vi "fpga_transmission_control_3V17.vi"() -> ()   [LabVIEW 2017]
doc: "3V15"
uses:
  Control 1.ctl
  <vilib>/Platform/TimedLoop/XDataNode/timing_clust.ctl
  <vilib>/Platform/TimedLoop/XDataNode/nitl_modes.ctl
  <vilib>/Platform/TimedLoop/XDataNode/wakeup.ctl
  <vilib>/Utility/config.llb/Read Key (String).vi
  <vilib>/Utility/config.llb/Write Key (String).vi
  <vilib>/Instr/_visa.llb/VISA Configure Serial Port (Serial Instr).vi
  <vilib>/platform/TimedLoop/XDataNode/XDataNode.xnode
  <vilib>/Platform/TimedLoop/XDataNode/XDNodeRunTimeDep.lvlib
  <vilib>/Utility/config.llb/NI_LVConfig.lvlib
  <vilib>/Analysis/NI_AALPro.lvlib
panel:
  in  "Tab Control":T1(tab)
  in  "Start":bool
  in  "Stop Program":bool
  out "Read":bool
  out "Sign":bool
  out "PWM":bool
  out "Output":bool
  out "Progress":dbl(slide) scale=0.0..100.0
  out "Time":dbl(slide) scale=0.0..100.0
  out "Timing":u32
  out "Timeslot":i32
  out "Timer":u32
  out "currentType":string
  out "Int_pixel":i16
  out "x-y":u16
  out "AD_Value":i16
  out "Complete Time":u32
  out "Kombi Chart":cluster{u16, i16}(graph)
  out "Histogram Graph":cluster{"Axis":dbl[], dbl[]}(graph)
  in  "fileName":string
  in  "pwmDtc":u8(slide)=25 scale=1.0..100.0
  in  "ExperimentalMetadata":T2
  in  "Fly":T3
  in  "Array":T5(array[cluster]) {"duration" step=1}
  in  "Path":path
  in  "VISA resource name":refnum<visa-resource-name>
  in  "LoadExperiment":bool
  in  "SaveExperiment":bool
  in  "ClearSetup":bool
  in  "Experimenter":T6
  in  "LoadMetadata":bool
  in  "SaveMetadata":bool
  in  "ClearMetaData":bool
  in  "URIs":T7
  out "VI Description":string
  out "outcome":u32
  in  "error in (no error)":errorcluster
  out "pattern":u32
  out "type":string
  out "contingency":string
  out "deleted portion":u8[](array[numeric])
  out "data":bool
  out "Error String":string
  out "error out":errorcluster
  in  "millisecond timer value 2":u32
  # "Universität Regensburg Elektronikwerkstatt Biologie/ VKL\n\njohann.schmid@ur.de"
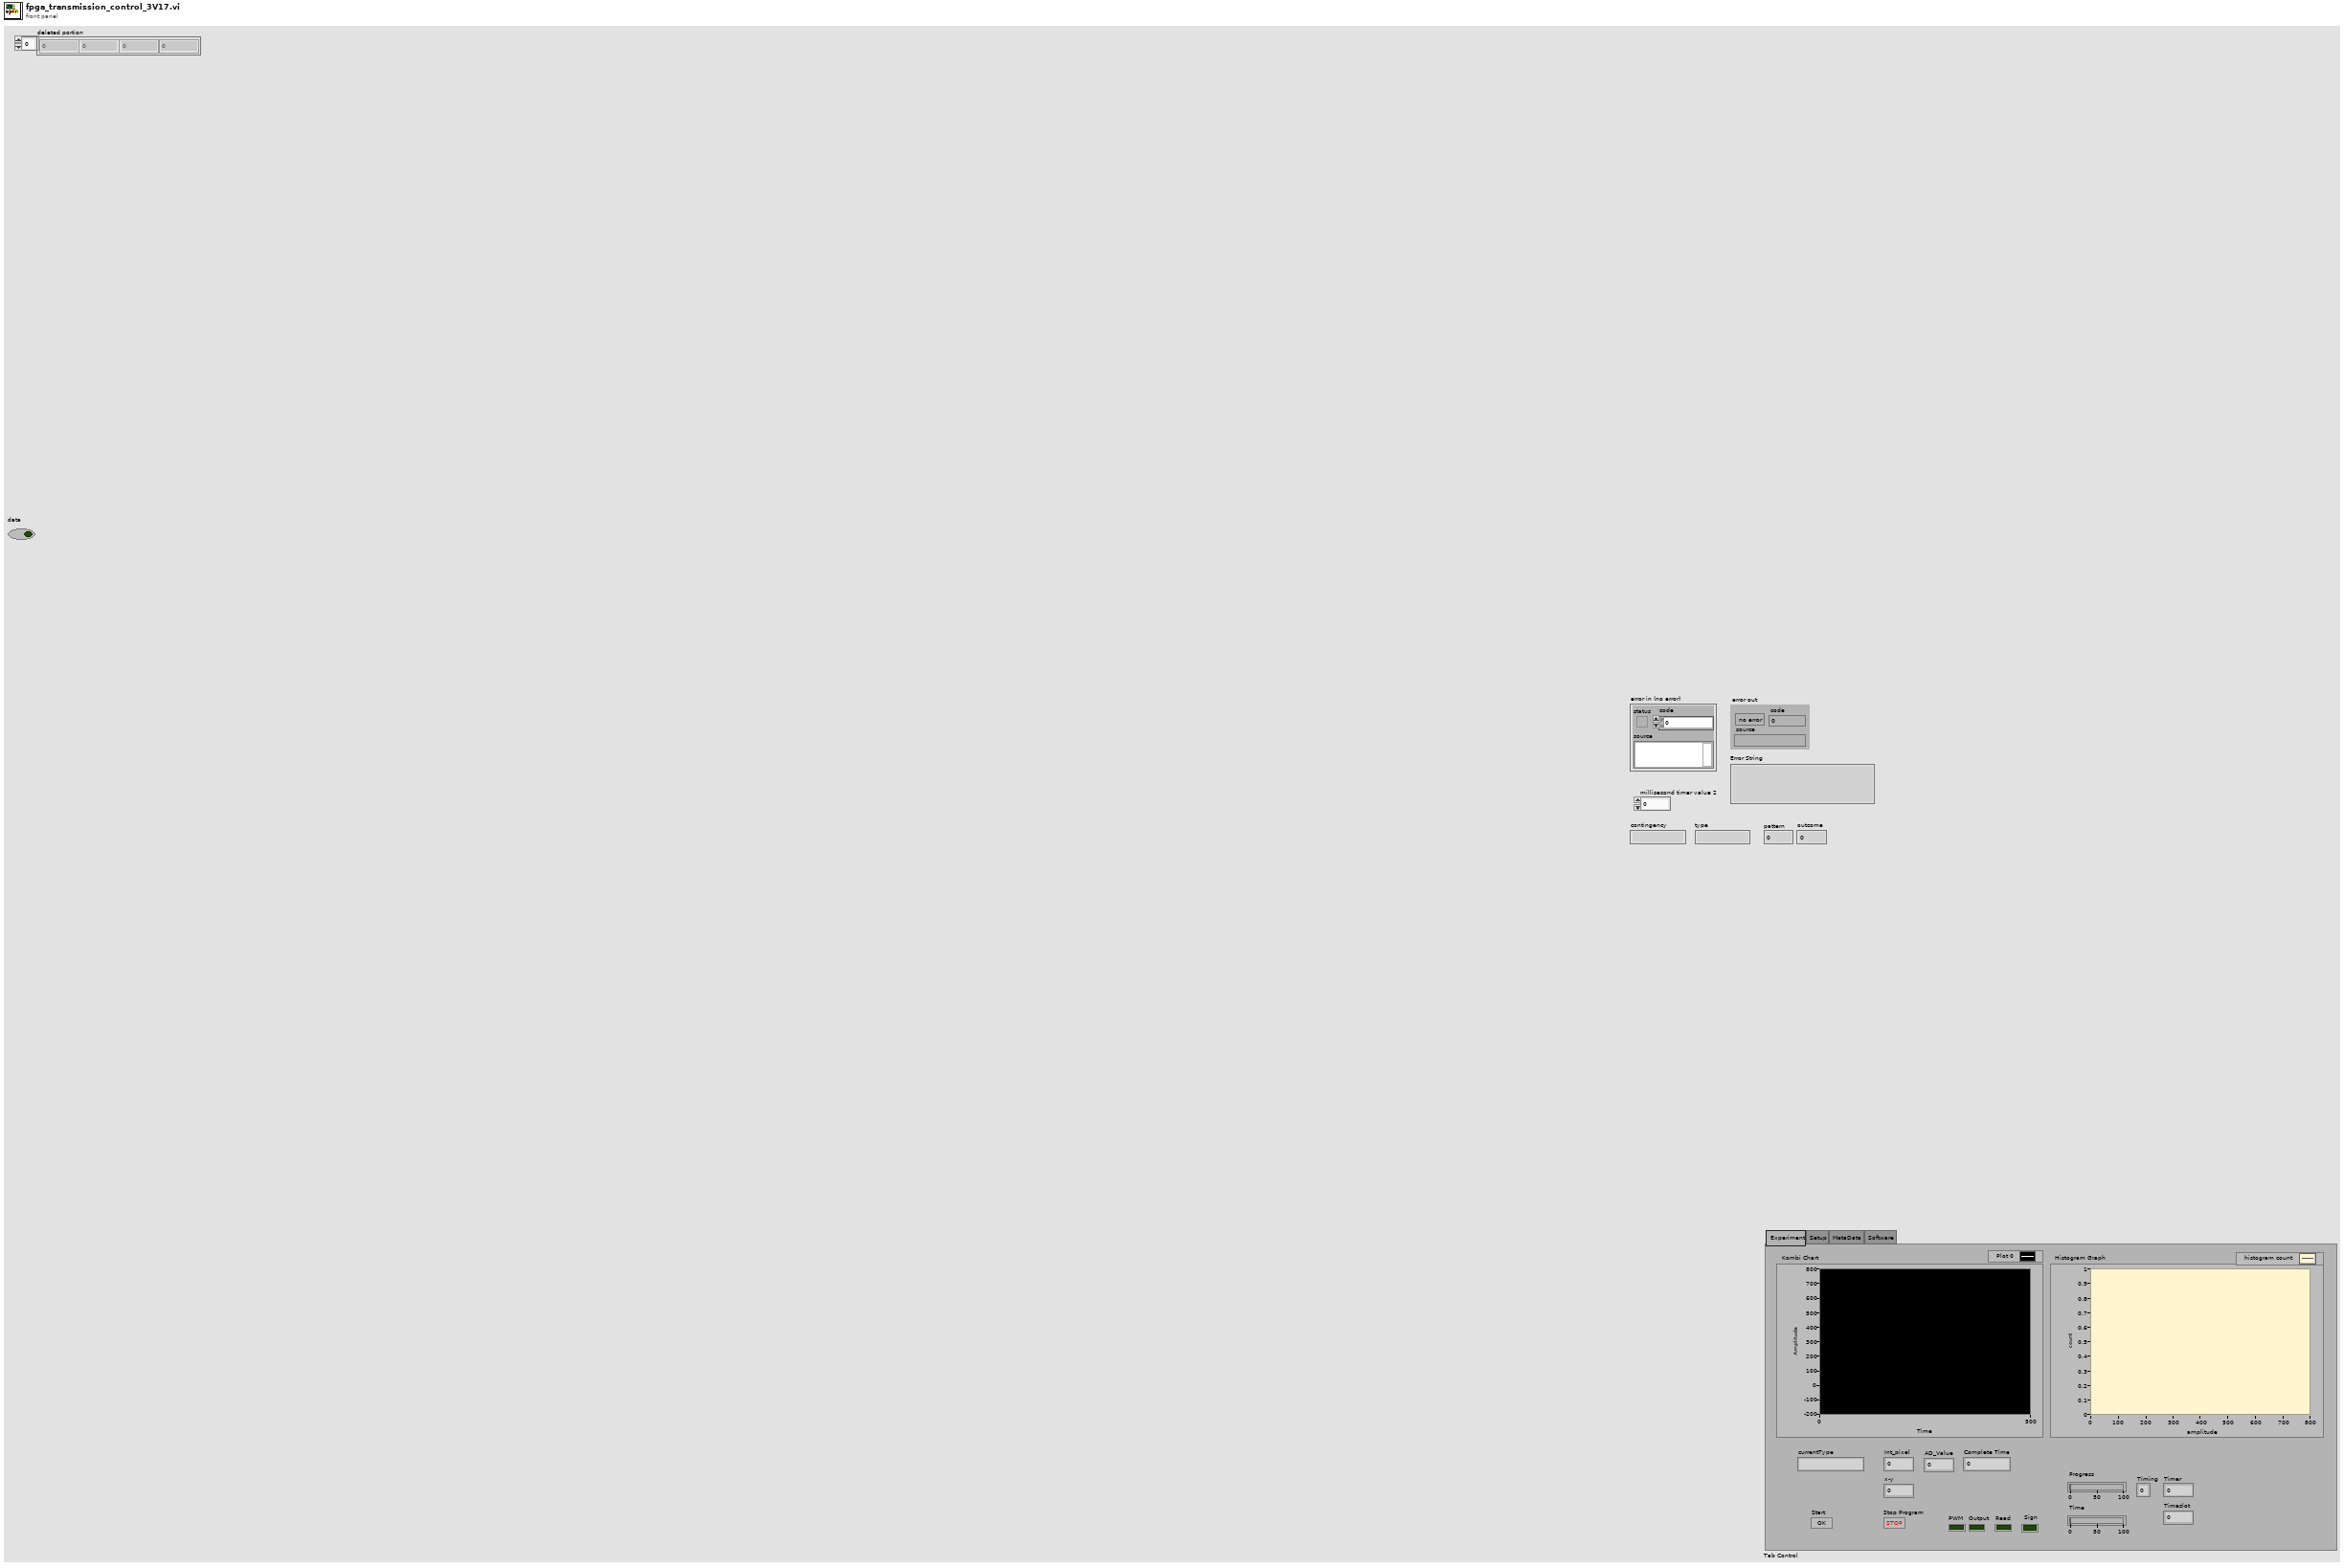
[diagram p1: front panel]
types:
  T1 = enum32{"Experiment", "Setup", "MetaData", "Software"}
  T2 = cluster{"Description":string, "ArenaType":string, "MeterType":string}
  T3 = cluster{"Name":string, "Description":string, "FlyBase":string, "f_parent":string, "m_parent":string}
  T4 = typedef "Control 1.ctl" = u32
  T5 = cluster{"type":string, "duration":T4, "outcome":u32, "pattern":u32, "coup_coeff":u32, "contingency":string}[]
  T6 = cluster{"FirstName":string, "LastName":string, "ORCID":string}
  T7 = cluster{"Recoding":string, "Analysis":string, "dataModel":string}
  T8 = typedef "XDNodeRunTimeDep.lvlib/timing_clust.ctl" = cluster{"Expected End [f-1]":u64, "Actual End [f-1]":u64, "Finished Late? [f-1]":bool, "Expected End [i-1]":u64, "Actual End [i-1]":u64, "Finished Late? [i-1]":bool, "Expected Start [i]":u64, "Actual Start [i]":u64, "Expected Start [f]":u64, "Actual Start [f]":u64, "Source Name":string, "Structure Name":string, "Period":i64, "Deadline":i64, "Offset":i64, "Start":i64, "Priority":i32, "Timeout":i32, "Mode":T9, "Wakeup Reason":T10, "Error":errorcluster, "Source Type":string, "Secondary Source Type":string, "Global End Time":u64, "Global Start Time":u64, "Frame Duration":u64, "Iteration Duration":u64, "Assigned CPU":i32, "I/O Scan Engine Mode":u32}
  T9 = typedef "XDNodeRunTimeDep.lvlib/nitl_modes.ctl" = enum32{"No Change", "Process missed periods, maintain original phase", "Discard missed periods, maintain original phase", "Process missed periods, ignore original phase", "Discard missed periods, ignore original phase"}
  T10 = typedef "XDNodeRunTimeDep.lvlib/wakeup.ctl" = enum32{"Normal", "Aborted", "Asynchronous wakeup", "Timing source error", "Timed loop error", "Timeout"}
  T11 = cluster{"String":string, i32, i32, u32, u32, "String":string}[]
  T12 = typedef "NI_LVConfig.lvlib/Config Data RefNum.ctl" = refnum<k1>
  T13 = cluster{"[0]":string, "[1]":string, "[2]":string, "[3]":string, "[4]":string}
  T14 = cluster{"[0]":string, "[1]":string, "[2]":string}
  T15 = cluster{"type":string, "duration":T4, "outcome":u32, "pattern":u32, "coup_coeff":u32, "contingency":string}
  T16 = enum16{"Idel", "State1", "State2", "State3", "State4"}
  T17 = enum16{"open", "replace", "create", "open or create", "replace or create", "replace or create with confirmation"}
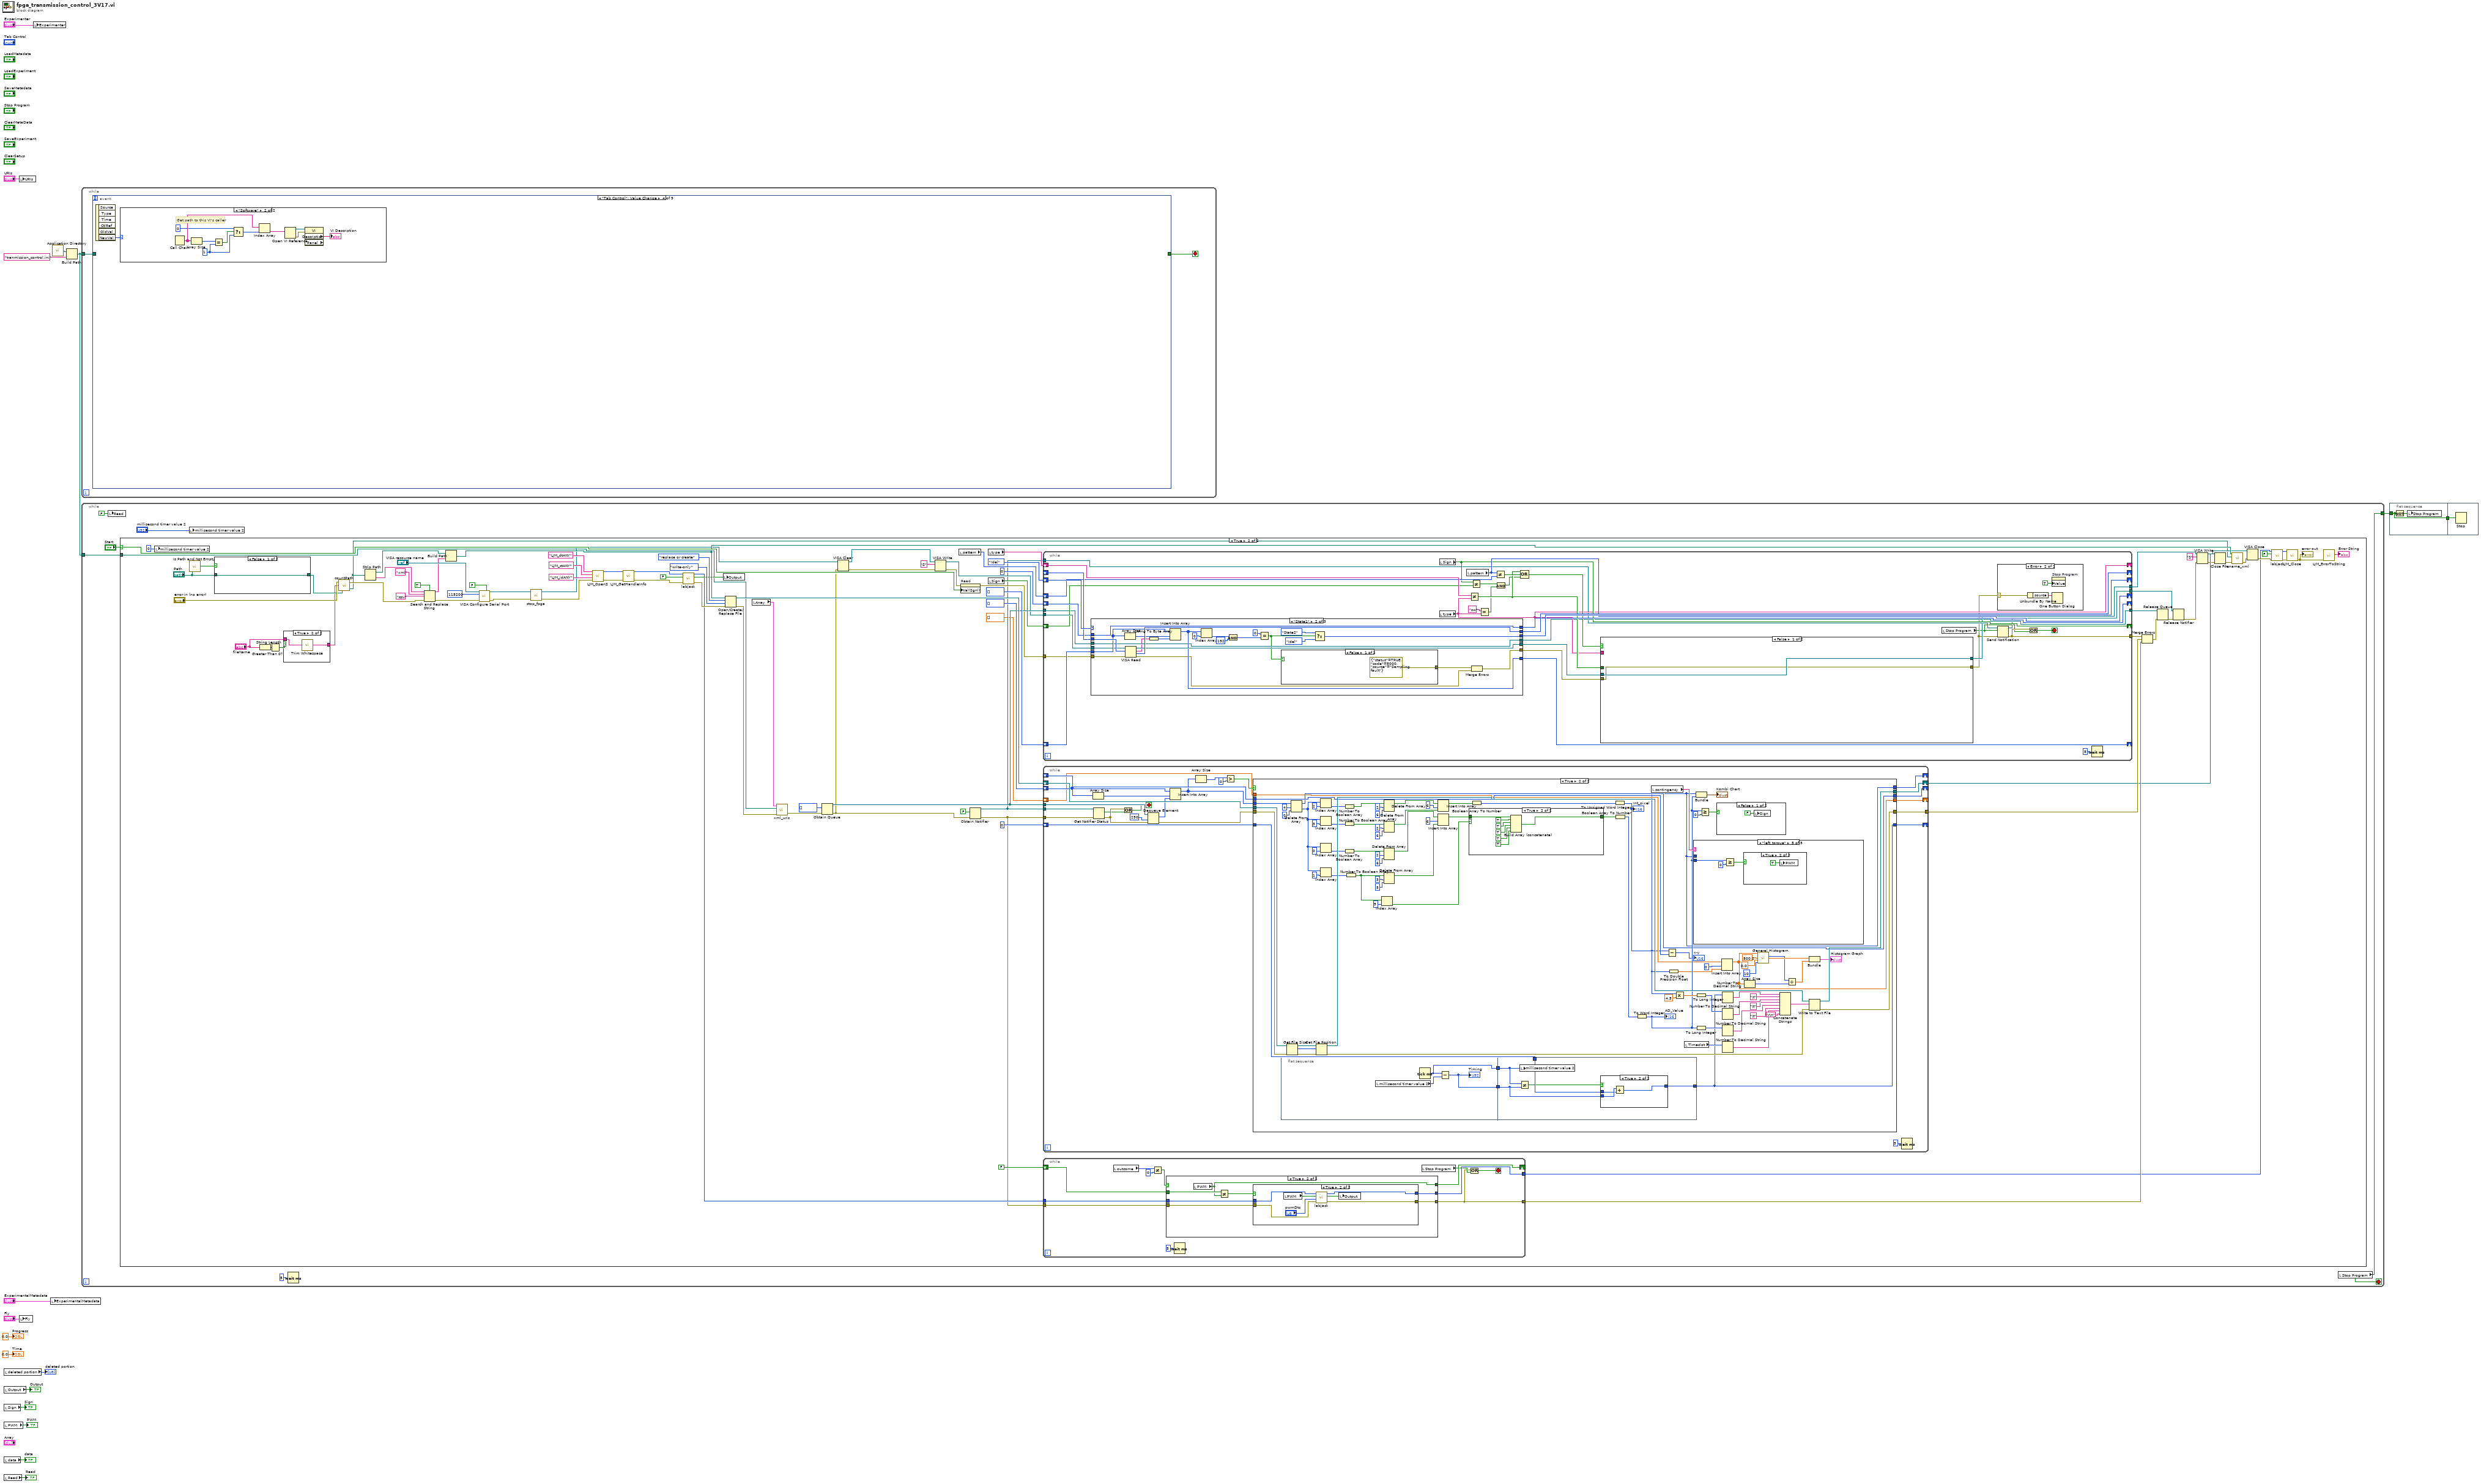
[diagram p0: block diagram]
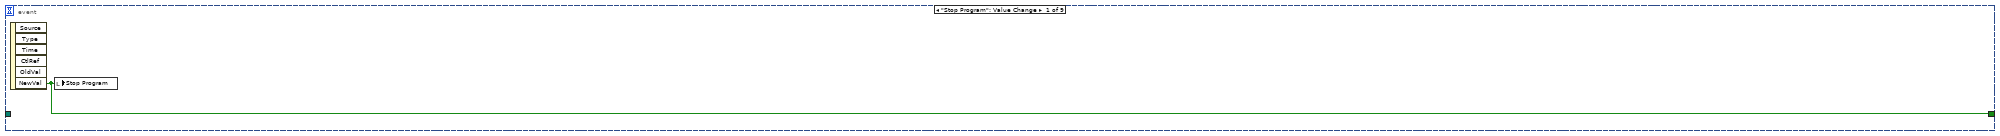
[diagram p2: hidden frame]
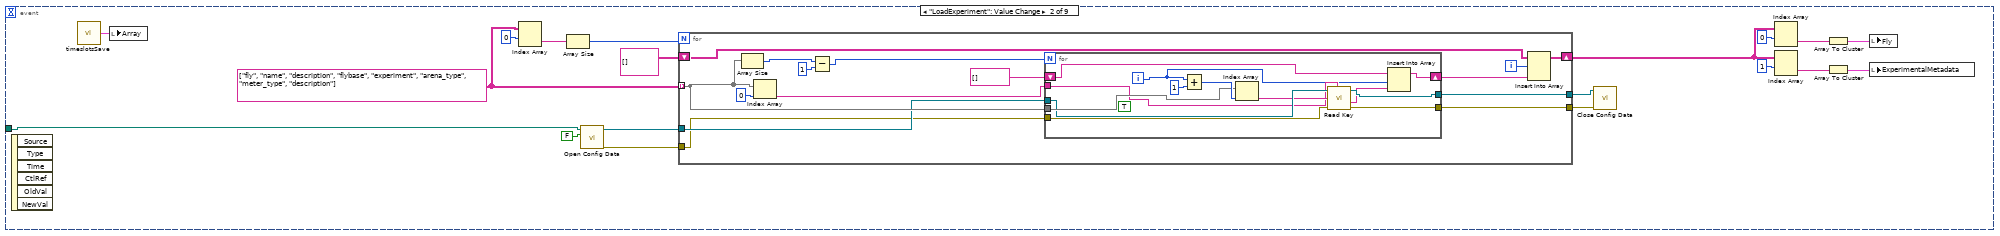
[diagram p3: hidden frame]
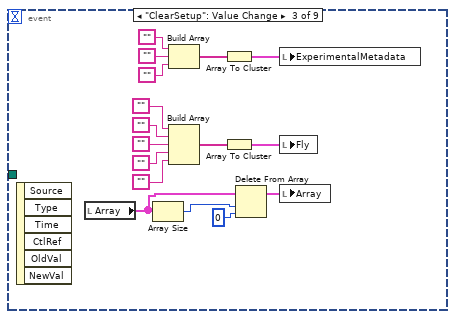
[diagram p4: hidden frame]
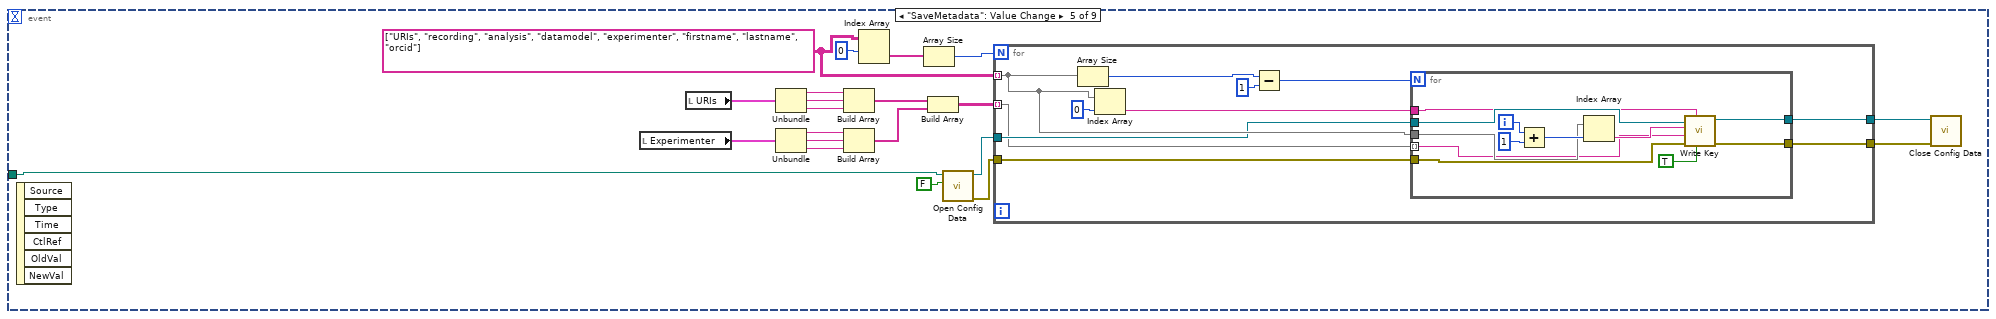
[diagram p6: hidden frame]
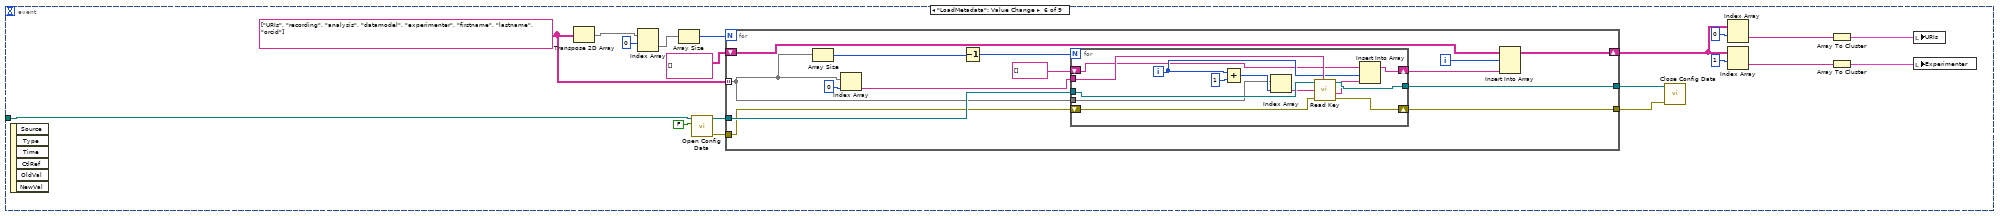
[diagram p7: hidden frame]
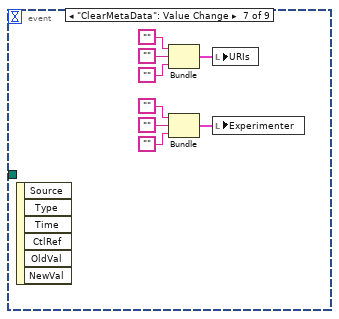
[diagram p8: hidden frame]
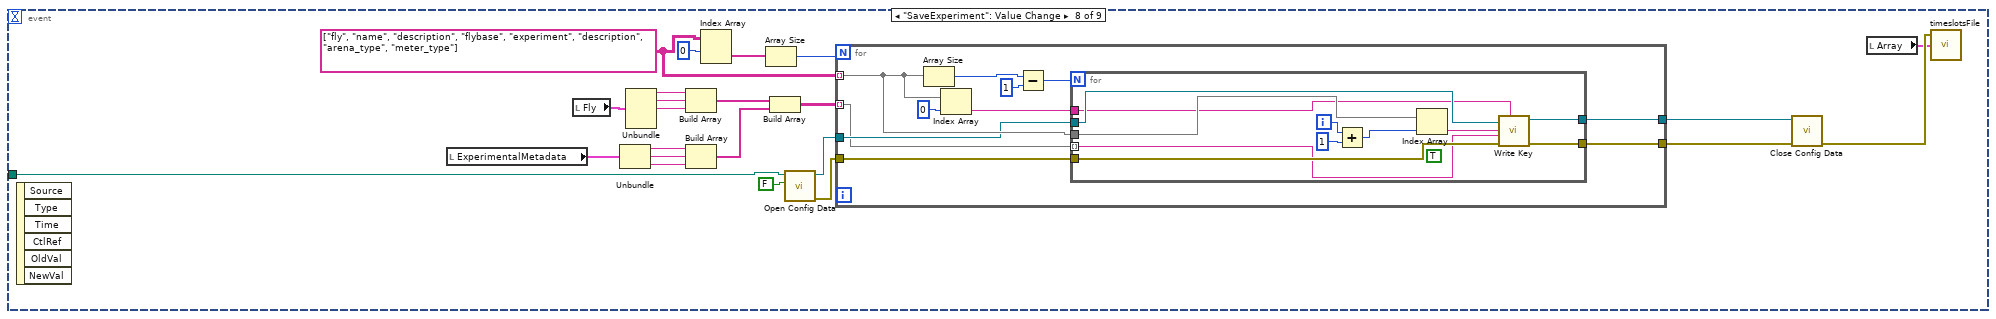
[diagram p9: hidden frame]
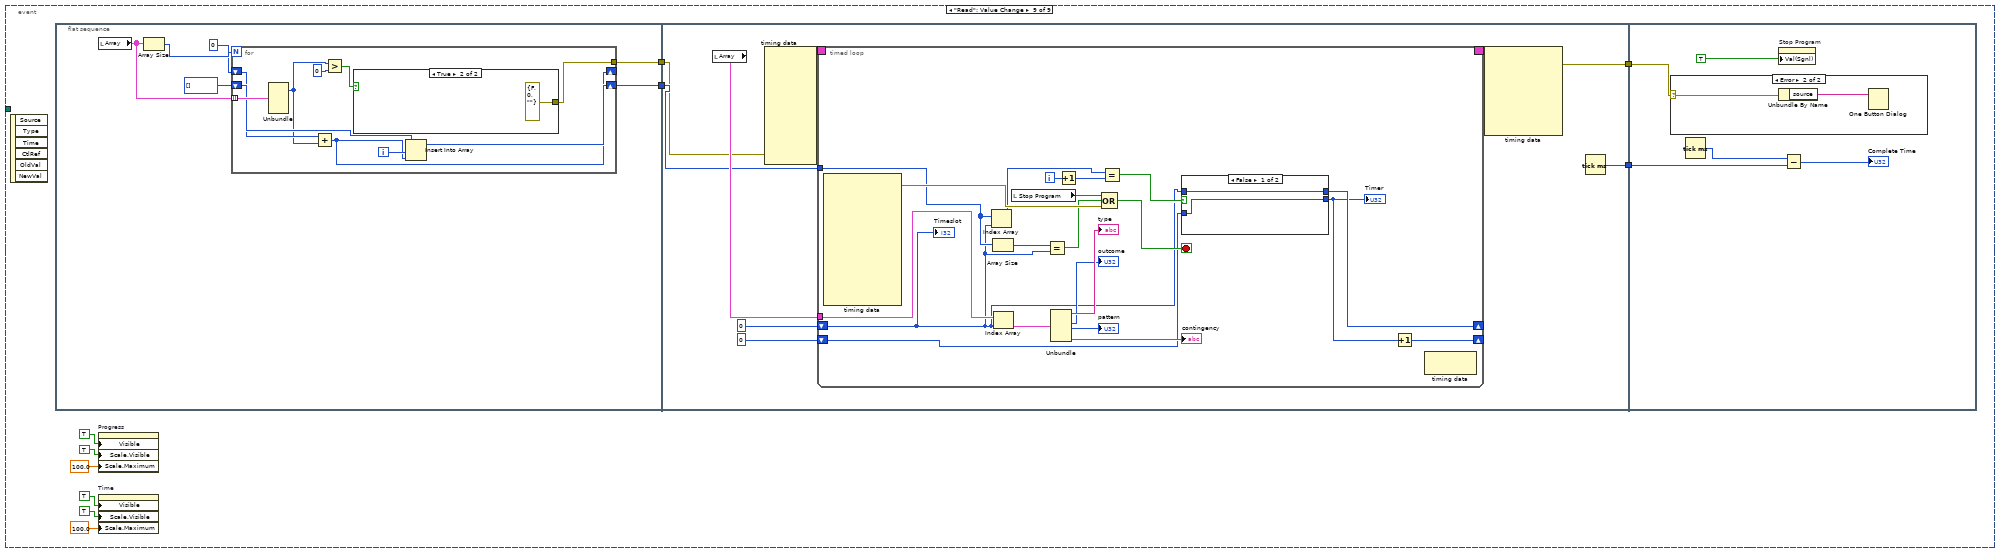
[diagram p10: hidden frame]
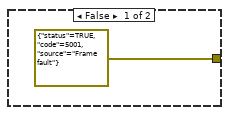
[diagram p11: hidden frame]
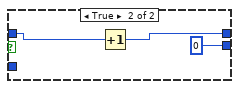
[diagram p12: hidden frame]
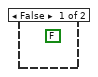
[diagram p14: hidden frame]
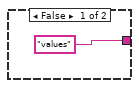
[diagram p15: hidden frame]
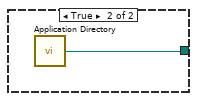
[diagram p16: hidden frame]
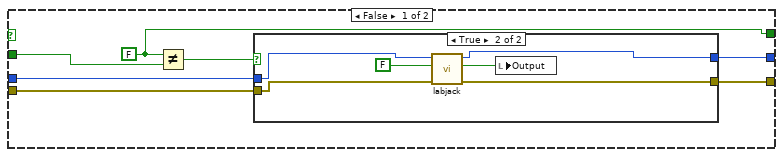
[diagram p17: hidden frame]
diagram:
  n1 = local read "deleted portion"() -> (→"deleted portion":u8[])
  n2 = local read "Output"() -> (→"Output":bool)
  n3 = local read "Sign"() -> (→"Sign":bool)
  n4 = local read "PWM"() -> (→"PWM":bool)
  n5 = local read "data"() -> (→"data":bool)
  n6 = local read "Read"() -> (→"Read":bool)
  n7 = local write "URIs"("URIs") -> ()
  n8 = local write "Fly"("Fly") -> ()
  n9 = local write "Experimenter"("Experimenter") -> ()
  n10 = local write "ExperimentalMetadata"("ExperimentalMetadata") -> ()
  n11 = call <vilib>:"Application Directory.vi"() -> ("Application Directory"=w5:path)
  n12 = Build Path(base path=w5, name or relative path="tranmission_control.ini") -> (appended path=w3:path)
  n13 = while {
    tunnel: w3 -> [w18]
    stop <- w19 stop-if-true
    n14 = event shown="[3] \"Tab Control\": Value Change" {
      selector: _ -> [_ _ _ _ _ _ _ _ _]
      dyn-events: _ -> [_ _ _ _ _ _ _ _ _]
      timeout: _ -> [_ _ _ _ _ _ _ _ _]
      tunnel: [w20 _ _ _ _ _ _ _ _] -> w19
      tunnel: w18 -> [_ w30 _ _ w95 w139 _ w195 _]
      event "Stop Program": Value Change {
        n15 = event-data() -> ("NewVal"=w20:bool)  [unwired: 1 in, 5 out]
        n16 = local write "Stop Program"(w20) -> ()
      }
      event "LoadExperiment": Value Change {
        w31 = string[][] [["fly", "name", "description", "flybase"], ["experiment", "arena_type", "meter_type", "description"]]
        n17 = event-data() -> ()  [unwired: 1 in, 6 out]
        n18 = call "timeslotsSave.vi"() -> ("array of clusters"=w39:T11)  [unwired: 1 in, 1 out]
        n19 = local write "Array"(w39) -> ()
        n20 = Index Array(array=w31, index (row)=0) -> (element=w36:string[])  [unwired: 1 in]
        n21 = Array Size(array=w36) -> (size(s)=w35:i32)
        n22 = call <vilib>:"Open Config Data.vi"("create file if necessary (T)"=FALSE, "configuration file path"=w30) -> ("error out"=w33:errorcluster, "refnum"=w34:T12)  [unwired: 7 in, 1 out]
        n23 = for {
          N: w35 -> [_]
          tunnel: w31 -> [w50] mode=indexing
          tunnel: w34 -> [w49]
          tunnel: w33 -> [w48]
          tunnel: [w46] -> w32
          tunnel: [w44] -> w29
          shift-right: [w42] -> w24
          shift-left: string[][] [] -> [w43]
          i -> [w40]
          n24 = Array Size(array=w50) -> (size(s)=w53:i32)
          n25 = Index Array(array=w50, index=0) -> (element=w47:string)
          n26 = Subtract(x=w53, y=1) -> (x-y=w51:i32)
          n27 = for {
            N: w51 -> [_]
            tunnel: w50 -> [w65]
            tunnel: w49 -> [w64]
            tunnel: w48 -> [w63]
            tunnel: w47 -> [w61]
            tunnel: [w60] -> w46
            shift-right: [w58] -> w41
            shift-left: string[] [] -> [w57]
            tunnel: [w59] -> w44
            i -> [w55]
            (unwired) TRUE ("write raw string? (F)")
            n28 = Add(x=w55, y=1) -> (x+y=w66:i32)
            n29 = Index Array(array=w65, index=w66) -> (element=w62:string)
            n30 = call-poly <vilib>:"Read Key.vi"("section"=w61, "error in (no error)"=w63, "key"=w62, "refnum"=w64) -> ("error out"=w59:errorcluster, "value"=w56:string, "refnum out"=w60:T12)  [unwired: 4 in, 1 out]
            n31 = Insert Into Array(array=w57, index=w55, new element=w56) -> (w58:string[])
          }
          n32 = Insert Into Array(array=w43, index (row)=w40, new element=w41) -> (w42:string[][])  [unwired: 1 in]
        }
        n33 = call <vilib>:"Close Config Data.vi"("error in (no error)"=w29, "refnum"=w32) -> ()  [unwired: 8 in, 2 out]
        n34 = Index Array(array=w24, index (row)=0) -> (element=w26:string[])  [unwired: 1 in]
        n35 = Index Array(array=w24, index (row)=1) -> (element=w22:string[])  [unwired: 1 in]
        n36 = Array To Cluster(array=w26) -> (cluster=w25:T13)
        n37 = Array To Cluster(array=w22) -> (cluster=w21:T14)
        n38 = local write "Fly"(w25) -> ()
        n39 = local write "ExperimentalMetadata"(w21) -> ()
      }
      event "ClearSetup": Value Change {
        n40 = event-data() -> ()  [unwired: 1 in, 6 out]
        n41 = local read "Array"() -> (w71:T5)
        n42 = Array Size(array=w71) -> (size(s)=w70:i32)
        n43 = Build Array("", "", "") -> (w76:string[])
        n44 = Build Array("", "", "", "", "") -> (w78:string[])
        n45 = Array To Cluster(array=w76) -> (cluster=w75:T14)
        n46 = Array To Cluster(array=w78) -> (cluster=w77:T13)
        n47 = Delete From Array(array=w71, length=w70, index=0) -> (array with subset deleted=w68:T5)  [unwired: 1 out]
        n48 = local write "ExperimentalMetadata"(w75) -> ()
        n49 = local write "Fly"(w77) -> ()
        n50 = local write "Array"(w68) -> ()
      }
      event "Tab Control": Value Change {
        n51 = event-data() -> ("NewVal"=w84:T1)  [unwired: 1 in, 5 out]
        n52 = case shown="\"Software\"" w84 {
          frame "Experiment", Default {
          }
          frame "Software" {
            w87 = 1 ("index")
            # "Get path to this VI's caller"
            n53 = Call Chain() -> (call chain=w88:string[])
            n54 = Array Size(array=w88) -> (size(s)=w91:i32)
            n55 = Equal?(x=w91, y=w87) -> (x = y?=w89:bool)
            n56 = Select(t=0, s=w89, f=w87) -> (s? t:f=w90:i32)
            n57 = Index Array(array=w88, index=w90) -> (element=w93:string)
            n58 = Open VI Reference(vi path=w93) -> (vi reference=w85:refnum<vi>, error out=w92:errorcluster)  [unwired: 5 in]
            n59 = property on="Property Node" class="VI" props=["Description", "Panel"](reference=w85, error in=w92) -> ("Description"=→"VI Description":string)  [unwired: 3 out]
          }
        }
      }
      event "SaveMetadata": Value Change {
        w111 = string[][] [["URIs", "recording", "analysis", "datamodel"], ["experimenter", "firstname", "lastname", "orcid"]]
        n60 = event-data() -> ()  [unwired: 1 in, 6 out]
        n61 = local read "Experimenter"() -> (w105:T6)
        n62 = local read "URIs"() -> (w104:T7)
        n63 = Unbundle(w104) -> ("Recoding"=w100:string, "Analysis"=w99:string, "dataModel"=w98:string)
        n64 = Unbundle(w105) -> ("FirstName"=w103:string, "LastName"=w102:string, "ORCID"=w101:string)
        n65 = Build Array(w100, w99, w98) -> (w97:string[])
        n66 = Build Array(w103, w102, w101) -> (w96:string[])
        n67 = Index Array(array=w111, index (row)=0) -> (element=w113:string[])  [unwired: 1 in]
        n68 = Array Size(array=w113) -> (size(s)=w112:i32)
        n69 = Build Array(w97, w96) -> (w106:string[][])
        n70 = call <vilib>:"Open Config Data.vi"("create file if necessary (T)"=FALSE, "configuration file path"=w95) -> ("error out"=w109:errorcluster, "refnum"=w110:T12)  [unwired: 7 in, 1 out]
        n71 = for {
          N: w112 -> [_]
          tunnel: w111 -> [w122] mode=indexing
          tunnel: w110 -> [w121]
          tunnel: w109 -> [w120]
          tunnel: [w118] -> w108
          tunnel: [w117] -> w107
          tunnel: w106 -> [w116] mode=indexing
          n72 = Array Size(array=w122) -> (size(s)=w125:i32)
          n73 = Index Array(array=w122, index=0) -> (element=w119:string)
          n74 = Subtract(x=w125, y=1) -> (x-y=w123:i32)
          n75 = for {
            N: w123 -> [_]
            tunnel: w122 -> [w136]
            tunnel: w121 -> [w135]
            tunnel: w120 -> [w134]
            tunnel: w119 -> [w132]
            tunnel: [w131] -> w118
            tunnel: [w130] -> w117
            tunnel: w116 -> [w128] mode=indexing
            i -> [w129]
            n76 = Add(x=w129, y=1) -> (x+y=w137:i32)
            n77 = Index Array(array=w136, index=w137) -> (element=w133:string)
            n78 = call-poly <vilib>:"Write Key.vi"("write raw string? (F)"=TRUE, "section"=w132, "error in (no error)"=w134, "value"=w128, "key"=w133, "refnum"=w135) -> ("error out"=w131:errorcluster, "refnum out"=w130:T12)  [unwired: 3 in, 1 out]
          }
        }
        n79 = call <vilib>:"Close Config Data.vi"("error in (no error)"=w108, "refnum"=w107) -> ()  [unwired: 8 in, 2 out]
      }
      event "LoadMetadata": Value Change {
        w149 = string[][] [["URIs", "recording", "analysis", "datamodel"], ["experimenter", "firstname", "lastname", "orcid"]]
        n80 = event-data() -> ()  [unwired: 1 in, 6 out]
        n81 = Transpose 2D Array(2D array=w149) -> (transposed array=w150:string[][])
        n82 = Index Array(array=w150, index (row)=0) -> (element=w155:string[])  [unwired: 1 in]
        n83 = Array Size(array=w155) -> (size(s)=w154:i32)
        n84 = call <vilib>:"Open Config Data.vi"("create file if necessary (T)"=FALSE, "configuration file path"=w139) -> ("error out"=w152:errorcluster, "refnum"=w153:T12)  [unwired: 7 in, 1 out]
        n85 = for {
          N: w154 -> [_]
          tunnel: w149 -> [w162] mode=indexing
          tunnel: w153 -> [w171]
          tunnel: w152 -> [w170]
          tunnel: [w169] -> w148
          tunnel: [w168] -> w147
          shift-right: [w161] -> w144
          shift-left: string[][] [] -> [w160]
          i -> [w159]
          n86 = Array Size(array=w162) -> (size(s)=w165:i32)
          n87 = Index Array(array=w162, index=0 ("index (row)")) -> (element=w166:string)
          n88 = Decrement(x=w165) -> (x-1=w164:i32)
          n89 = for {
            N: w164 -> [_]
            shift-right: [w179] -> w168
            shift-left: w170 -> [w181]
            tunnel: w166 -> [w178]
            tunnel: w171 -> [w182]
            tunnel: [w180] -> w169
            shift-right: [w175] -> w158
            shift-left: string[] [] -> [w174]
            tunnel: w162 -> [w173]
            i -> [w176]
            n90 = Add(x=w176, y=1) -> (x+y=w184:i32)
            n91 = Index Array(array=w173, index=w184) -> (element=w172:string)
            n92 = call-poly <vilib>:"Read Key.vi"("section"=w178, "error in (no error)"=w181, "key"=w172, "refnum"=w182) -> ("error out"=w179:errorcluster, "value"=w177:string, "refnum out"=w180:T12)  [unwired: 4 in, 1 out]
            n93 = Insert Into Array(array=w174, index=w176, new element=w177) -> (w175:string[])
          }
          n94 = Insert Into Array(array=w160, index (row)=w159, new element=w158) -> (w161:string[][])  [unwired: 1 in]
        }
        n95 = call <vilib>:"Close Config Data.vi"("error in (no error)"=w147, "refnum"=w148) -> ()  [unwired: 8 in, 2 out]
        n96 = Index Array(array=w144, index (row)=0) -> (element=w141:string[])  [unwired: 1 in]
        n97 = Index Array(array=w144, index (row)=1) -> (element=w143:string[])  [unwired: 1 in]
        n98 = Array To Cluster(array=w141) -> (cluster=w140:T14)
        n99 = Array To Cluster(array=w143) -> (cluster=w142:T14)
        n100 = local write "URIs"(w140) -> ()
        n101 = local write "Experimenter"(w142) -> ()
      }
      event "ClearMetaData": Value Change {
        n102 = event-data() -> ()  [unwired: 1 in, 6 out]
        n103 = Bundle("", "", "") -> (w192:cluster{string, string, string})  [unwired: 1 in]
        n104 = Bundle("", "", "") -> (w191:cluster{string, string, string})  [unwired: 1 in]
        n105 = local write "URIs"(w192) -> ()
        n106 = local write "Experimenter"(w191) -> ()
      }
      event "SaveExperiment": Value Change {
        w203 = string[][] [["fly", "name", "description", "flybase"], ["experiment", "description", "arena_type", "meter_type"]]
        n107 = event-data() -> ()  [unwired: 1 in, 6 out]
        n108 = local read "ExperimentalMetadata"() -> (w202:T2)
        n109 = local read "Fly"() -> (w207:T3)
        n110 = Unbundle(w202) -> ("Description"=w201:string, "ArenaType"=w200:string, "MeterType"=w199:string)
        n111 = Unbundle(w207) -> ("Name"=w206:string, "Description"=w205:string, "FlyBase"=w204:string)  [unwired: 2 out]
        n112 = Build Array(w206, w205, w204) -> (w198:string[])
        n113 = Build Array(w201, w200, w199) -> (w197:string[])
        n114 = Index Array(array=w203, index (row)=0) -> (element=w213:string[])  [unwired: 1 in]
        n115 = Array Size(array=w213) -> (size(s)=w212:i32)
        n116 = Build Array(w198, w197) -> (w196:string[][])
        n117 = call <vilib>:"Open Config Data.vi"("create file if necessary (T)"=FALSE, "configuration file path"=w195) -> ("error out"=w210:errorcluster, "refnum"=w211:T12)  [unwired: 7 in, 1 out]
        n118 = for {
          N: w212 -> [_]
          tunnel: w203 -> [w222] mode=indexing
          tunnel: w211 -> [w221]
          tunnel: w210 -> [w220]
          tunnel: [w218] -> w209
          tunnel: [w217] -> w208
          tunnel: w196 -> [w216] mode=indexing
          n119 = Array Size(array=w222) -> (size(s)=w225:i32)
          n120 = Index Array(array=w222, index=0) -> (element=w219:string)
          n121 = Subtract(x=w225, y=1) -> (x-y=w223:i32)
          n122 = for {
            N: w223 -> [_]
            tunnel: w222 -> [w235]
            tunnel: w221 -> [w234]
            tunnel: w220 -> [w233]
            tunnel: w219 -> [w231]
            tunnel: [w230] -> w218
            tunnel: [w229] -> w217
            tunnel: w216 -> [w227] mode=indexing
            i -> [w228]
            (unwired) TRUE ("write raw string? (F)")
            n123 = Add(x=w228, y=1) -> (x+y=w236:i32)
            n124 = Index Array(array=w235, index=w236) -> (element=w232:string)
            n125 = call-poly <vilib>:"Write Key.vi"("section"=w231, "error in (no error)"=w233, "value"=w227, "key"=w232, "refnum"=w234) -> ("error out"=w230:errorcluster, "refnum out"=w229:T12)  [unwired: 4 in, 1 out]
          }
        }
        n126 = call <vilib>:"Close Config Data.vi"("error in (no error)"=w209, "refnum"=w208) -> ("error out"=w194:errorcluster)  [unwired: 8 in, 1 out]
        n127 = local read "Array"() -> (w193:T5)
        n128 = call "timeslotsFile.vi"("array of clusters"=w193, "error in"=w194) -> ()  [unwired: 1 out]
      }
      event "Read": Value Change {
        n129 = event-data() -> ()  [unwired: 1 in, 6 out]
        n130 = flat-sequence {
          tunnel: [w249] -> w241
          tunnel: [w248] -> w240
          tunnel: w241 -> [w271]
          tunnel: w240 -> [w270]
          tunnel: [w269] -> w239
          tunnel: [w267] -> w238
          tunnel: w239 -> [w312]
          tunnel: w238 -> [w309]
          frame #0 {
            n131 = local read "Array"() -> (w252:T5)
            n132 = Array Size(array=w252) -> (size(s)=w253:i32)
            n133 = for {
              N: w253 -> [_]
              tunnel: w252 -> [w263] mode=indexing
              shift-right: [w261] -> w249
              shift-left: T4[] [] -> [w260]
              shift-right: [w258] -> _
              shift-left: T4 0 ("duration") -> [w259]
              tunnel: [w254] -> w248
              i -> [w262]
              n134 = Unbundle(w263) -> ("duration"=w256:T4)  [unwired: 5 out]
              n135 = Add(x=w259, y=w256) -> (x+y=w258:T4)
              n136 = Greater?(x=w256, y=T4 0) -> (0:w257:bool)
              n137 = case shown="True" w257 {
                tunnel: [errorcluster {"status"=TRUE, "code"=5001, "source"="Frame fault"} ("error constant") errorcluster {"status"=FALSE, "code"=0, "source"=""} ("error constant")] -> w254
                frame False {
                }
                frame True {
                }
              }
              n138 = Insert Into Array(array=w260, index=w262, new element=w258) -> (w261:T4[])
            }
          }
          frame #1 {
            n139 = local read "Array"() -> (w272:T5)
            n140 = node-c288(w270) -> (w274:T8)  [unwired: 9 in]
            n141 = timed-loop {
              timing: w274 -> [_]
              timing-out: [_] -> w273
              tunnel: w272 -> [w290]
              tunnel: w271 -> [w284]
              shift-right: [w287] -> _
              shift-left: T4 0 ("duration") -> [w282]
              shift-right: [w277] -> _
              shift-left: 0 -> [w276]
              i -> [w279]
              stop <- w289 stop-if-true
              n142 = node-c288() -> (w288:errorcluster)  [unwired: 1 in, 11 out]
              n143 = Index Array(array=w284, index=w282) -> (element=w286:T4)
              n144 = Array Size(array=w284) -> (size(s)=w283:i32)
              n145 = Index Array(array=w290, index=w282) -> (element=w295:T15)
              n146 = local read "Stop Program"() -> (w281:bool)
              n147 = Equal?(x=w283, y=w282) -> (x = y?=w280:bool)
              n148 = Unbundle(w295) -> ("type"=→"type":string, "outcome"=→"outcome":u32, "pattern"=→"pattern":u32, "contingency"=→"contingency":string)  [unwired: 2 out]
              n149 = Increment(x=w279) -> (x+1=w278:i32)
              n150 = Equal?(x=w286, y=w278) -> (x = y?=w285:bool)
              n151 = Compound Arithmetic op=OR(w281, w280, w288) -> (w289:bool)
              n152 = case shown="False" w285 {
                tunnel: [w297 w300] -> w287
                tunnel: w282 -> [w297 w299]
                tunnel: w276 -> [w296 _]
                tunnel: [w296 0] -> w275
                frame False {
                }
                frame True {
                  n153 = Increment(x=w299) -> (x+1=w300:T4)
                }
              }
              "Timer" <- w275
              n154 = Increment(x=w275) -> (x+1=w277:i32)
              n155 = node-c288() -> ()  [unwired: 1 in, 1 out]
              "Timeslot" <- w282
            }
            n156 = node-c288(w273) -> (w269:errorcluster)  [unwired: 6 out]
            n157 = Tick Count (ms)() -> (millisecond timer value=w267:u32)
          }
          frame #2 {
            n158 = case shown="Error" w312 {
              selector: w312 -> [_ w315]
              frame No Error {
              }
              frame Error {
                n159 = Unbundle By Name(w315) -> ("source"=w314:string)
                n160 = One Button Dialog(message=w314) -> ()  [unwired: 1 in, 1 out]
              }
            }
            n161 = Tick Count (ms)() -> (millisecond timer value=w310:u32)
            n162 = property on="Stop Program" class="Bool (strict)"("Val(Sgnl)"=TRUE) -> ()  [unwired: 2 in, 2 out]
            n163 = Subtract(x=w310, y=w309) -> (x-y=→"Complete Time":u32)
          }
        }
        n164 = property on="Progress" class="Slide (strict)"("Visible"=TRUE, "Scale.Visible"=TRUE ("Visible"), "Scale.Maximum"=100.0 ("Scale.Range:Maximum")) -> ()  [unwired: 2 in, 2 out]
        n165 = property on="Time" class="Slide (strict)"("Visible"=TRUE, "Scale.Visible"=TRUE ("Visible"), "Scale.Maximum"=100.0 ("Scale.Range:Maximum")) -> ()  [unwired: 2 in, 2 out]
      }
    }
  }
  n166 = while {
    tunnel: [w320] -> w17
    tunnel: w3 -> [w316]
    stop <- w320 stop-if-true
    n167 = local write "Read"(FALSE) -> ()
    n168 = case shown="True" "Start" {
      selector: "Start" -> [_ w404]
      tunnel: w316 -> [_ w333]
      frame False {
        (unwired) FALSE
      }
      frame True {
        n169 = local write "millisecond timer value 2"(u32 0 ("millisecond timer value 2")) -> ()
        n170 = call <vilib>:"Is Path and Not Empty.vi"("path"="Path") -> ("Is Path and Not Empty?"=w323:bool)  [unwired: 4 in]
        n171 = case shown="False" w323 {
          tunnel: [w414 w415] -> w326
          tunnel: "Path" -> [w414 _]
          frame False {
          }
          frame True {
            n172 = call <vilib>:"Application Directory.vi"() -> ("Application Directory"=w415:path)
          }
        }
        n173 = String Length(string="fileName") -> (length=w330:i32)
        n174 = Greater Than 0?(x=w330) -> (x > 0?=w331:bool)
        n175 = case shown="True" w331 {
          tunnel: "fileName" -> [_ w413]
          tunnel: ["values" w412] -> w325
          frame False {
          }
          frame True {
            n176 = call <vilib>:"Trim Whitespace.vi"("string"=w413) -> ("trimmed string"=w412:string)  [unwired: 1 in]
          }
        }
        n177 = call "countPath.vi"("inputPath"=w326, "String"=w325, "error in (no error)"="error in (no error)") -> ("appended path"=w328:path, "error out"=w329:errorcluster)
        n178 = Strip Path(path=w328) -> (stripped path=w374:path, name=w373:string)
        n179 = Search and Replace String(case sensitive?=TRUE ("ignore case? (F)"), input string=w373, search string="xml", replace string="csv" ("replace string (\"\")"), error in=w329) -> (result string=w368:string, error out=w370:errorcluster)  [unwired: 3 in, 2 out]
        n180 = Build Path(base path=w374, name or relative path=w368) -> (appended path=w363:path)
        n181 = call-poly "VISA Configure Serial Port"("VISA resource name"="VISA resource name", "Enable Termination\nChar (T)"=FALSE ("Enable Termination\nChar (T)"), "baud rate (9600)"=u32 115200, "error in (no error)"=w370) -> ("VISA resource name out"=w356:refnum<visa-resource-name>, "error out"=w355:errorcluster)  [unwired: 10 in]
        n182 = call "stop_fpga.vi"("error in (no error)"=w355, "reference"=w356) -> ("error out"=w354:errorcluster, "VISA resource name out"=w347:refnum<visa-resource-name>)  [unwired: 2 in]
        n183 = call "LJM_OpenS.vi"("error in"=w354, "Identifier"="LJM_idANY", "ConnectionType"="LJM_ctANY", "DeviceType"="LJM_dtANY") -> ("error out"=w394:errorcluster, "Handle"=w393:i32)  [unwired: 6 in]
        n184 = call "LJM_GetHandleInfo.vi"("error in"=w394, "Handle In"=w393) -> ("error out"=w396:errorcluster, "Handle Out"=w395:i32)  [unwired: 2 in, 6 out]
        n185 = call "labjack.vi"("error out"=w396, "Boolean"=FALSE, "Handle Out"=w395) -> ("error out 2"=w399:errorcluster, "Boolean 2"=w362:bool, "Handle Out 2"=w398:i32)  [unwired: 6 in]
        n186 = local write "Output"(w362) -> ()
        n187 = Open/Create/Replace File(file path (use dialog)=w363, error in=w399, operation (0:open)=T17."replace or create", access (0:read/write)=enum16{"read/write", "read-only", "write-only"}."write-only") -> (refnum out=w377:refnum<file>, error out=w375:errorcluster)  [unwired: 2 in, 1 out]
        n188 = local read "Array"() -> (w376:T5)
        n189 = call "xml_uris.vi"("error in"=w375, "Path"=w333, "Array"=w376) -> ("error out"=w348:errorcluster)  [unwired: 1 in, 2 out]
        n190 = Obtain Queue(element data type=u8[] [], error in (no error)=w348) -> (queue out=w350:refnum<queue>, error out=w335:errorcluster)  [unwired: 3 in, 1 out]
        n191 = VISA Clear(VISA resource name=w347, error in (no error)=w335) -> (VISA resource name out=w346:refnum<visa-resource-name>, error out=w344:errorcluster)
        n192 = VISA Write(VISA resource name=w346, write buffer="S", error in (no error)=w344) -> (VISA resource name out=w345:refnum<visa-resource-name>, error out=w353:errorcluster)  [unwired: 1 out]
        n193 = local read "pattern"() -> (w379:u32)
        n194 = property on="Read" class="Bool (strict)"(error in=w353, "Val(Sgnl)"=w404) -> (error out=w343:errorcluster)  [unwired: 1 in, 1 out]
        n195 = Obtain Notifier(notification data type=FALSE, error in (no error)=w335) -> (notifier out=w341:refnum<notifier>, error out=w334:errorcluster)  [unwired: 2 in, 1 out]
        n196 = local read "type"() -> (w400:string)
        n197 = local read "Sign"() -> (w378:bool)
        n198 = while {
          tunnel: w345 -> [w676]
          shift-right: [w670] -> _
          shift-left: u8[] [] -> [w675]
          tunnel: [w652] -> w359
          shift-right: [w674] -> _
          shift-left: T16."Idel" -> [w673]
          shift-right: [w672] -> _
          shift-left: _ -> [w671]
          shift-right: [w669] -> _
          shift-left: u8 0 -> [w668]
          shift-right: [w659] -> _
          shift-left: w400 -> [w667]
          shift-right: [w666] -> _
          shift-left: w379 -> [w665]
          shift-right: [w664] -> _
          shift-left: w378 -> [w663]
          tunnel: w350 -> [w651]
          tunnel: [w650] -> w349
          tunnel: w341 -> [w647]
          tunnel: w343 -> [w648]
          tunnel: [w644] -> w338
          tunnel: [w645] -> w339
          stop <- w642 stop-if-true
          n199 = case shown="\"State1\"" w673 {
            tunnel: w676 -> [w794 w821 w839]
            tunnel: w648 -> [w795 w822 w833]
            tunnel: w675 -> [w798 w824 w846]
            tunnel: [w802 w825 w839] -> w653
            tunnel: [w801 w810 w832] -> w654
            tunnel: [w803 w823 w842] -> w674
            tunnel: [w800 w826 w840] -> w672
            tunnel: w671 -> [_ w827 w840]
            tunnel: [w798 w820 w845] -> w670
            tunnel: [w797 w819 u8 0] -> w669
            tunnel: w668 -> [w797 w819 _]
            tunnel: w651 -> [w792 w813 w835]
            tunnel: [w792 w813 w834] -> w650
            frame "Idel", Default {
              n200 = local write "data"(FALSE ("data")) -> ()
              n201 = property class="Serial Instr"(reference=w794, error in=w795) -> (reference out=w802:refnum<visa-resource-name>, error out=w801:errorcluster, "Serial Settings:Number of Bytes at Serial Port"=w800:u32)
              n202 = Greater Or Equal?(x=w800, y=u8 4) -> (x >= y?=w793:bool)
              n203 = Select(t=T16."State1", s=w793, f=T16."Idel") -> (s? t:f=w803:T16)
            }
            frame "State1" {
              n204 = Array Size(array=w824) -> (size(s)=w812:i32)
              n205 = VISA Read(VISA resource name=w821, byte count=w827, error in (no error)=w822) -> (VISA resource name out=w825:refnum<visa-resource-name>, read buffer=w807:string, return count=w826:u32, error out=w808:errorcluster)
              n206 = String To Byte Array(string=w807) -> (unsigned byte array=w806:u8[])
              n207 = Insert Into Array(array=w824, index=w812, new element=w806) -> (w820:u8[])
              n208 = Index Array(array=w820, index=0) -> (element=w817:u8)
              n209 = And(x=w817, y=u8 192) -> (x .and. y?=w816:u8)
              n210 = Equal?(x=u8 0, y=w816) -> (x = y?=w809:bool)
              n211 = case shown="False" w809 {
                tunnel: [errorcluster {"status"=TRUE, "code"=5000, "source"="Sampling fault"} ("error constant") errorcluster {"status"=FALSE, "code"=0, "source"=""} ("error constant")] -> w811
                frame False {
                }
                frame True {
                }
              }
              n212 = Select(t=T16."State2", s=w809, f=T16."Idel") -> (s? t:f=w823:T16)
              n213 = Merge Errors(w811, w808) -> (w810:errorcluster)
            }
            frame "State2" {
              n214 = Delete From Array(array=w846, length=4, index=0) -> (deleted portion=w836:u8[], array with subset deleted=w845:u8[])
              n215 = Array Size(array=w845) -> (size(s)=w844:i32)
              n216 = Enqueue Element(queue=w835, element=w836, error in (no error)=w833) -> (queue out=w834:refnum<queue>, error out=w832:errorcluster)  [unwired: 1 in, 1 out]
              n217 = Greater Or Equal?(x=w844, y=4) -> (x >= y?=w837:bool)
              n218 = Select(t=T16."State2", s=w837, f=T16."Idel") -> (s? t:f=w842:T16)
            }
          }
          n219 = local read "Sign"() -> (w664:bool)
          n220 = local read "type"() -> (w659:string)
          n221 = local read "pattern"() -> (w666:u32)
          n222 = Not Equal?(x=w667, y=w659) -> (x != y?=w660:bool)
          n223 = Not Equal?(x=w664, y=w663) -> (x != y?=w656:bool)
          n224 = Equal?(x="sw", y=w659) -> (x = y?=w657:bool)
          n225 = Not Equal?(x=w666, y=w665) -> (x != y?=w662:bool)
          n226 = And(x=w656, y=w657) -> (x .and. y?=w655:bool)
          n227 = Compound Arithmetic op=OR(w660, w662, w655) -> (w661:bool)
          n228 = case shown="False" w661 {
            tunnel: w653 -> [w681 w685]
            tunnel: [w681 w688] -> w652
            tunnel: w654 -> [w680 w684]
            tunnel: [w680 w689] -> w646
            tunnel: w659 -> [_ w682]
            tunnel: w660 -> [_ w683]
            frame False {
            }
            frame True {
              n229 = case shown="True" w683 {
                tunnel: [w691 w697] -> w687
                tunnel: [w692 w696] -> w686
                tunnel: w685 -> [w692 w694]
                tunnel: w684 -> [w691 w693]
                frame False {
                }
                frame True {
                  n230 = VISA Write(VISA resource name=w694, write buffer="1W", error in (no error)=w693) -> (VISA resource name out=w696:refnum<visa-resource-name>, error out=w697:errorcluster)  [unwired: 1 out]
                }
              }
              n231 = case shown="\"fs\"" w682 {
                tunnel: w686 -> [w699 w706 w711 w719 w730 w767]
                tunnel: [w701 w705 w710 w713 w729 w766] -> w688
                tunnel: w687 -> [w698 w704 w709 w718 w732 w769]
                tunnel: [w700 w703 w708 w714 w731 w768] -> w690
                frame "False", Default {
                  n232 = VISA Write(VISA resource name=w699, write buffer="s4s", error in (no error)=w698) -> (VISA resource name out=w701:refnum<visa-resource-name>, error out=w700:errorcluster)  [unwired: 1 out]
                }
                frame "optomotorR" {
                  n233 = VISA Write(VISA resource name=w706, write buffer="s3r", error in (no error)=w704) -> (VISA resource name out=w705:refnum<visa-resource-name>, error out=w703:errorcluster)  [unwired: 1 out]
                }
                frame "optomotorL" {
                  n234 = VISA Write(VISA resource name=w711, write buffer="s3l", error in (no error)=w709) -> (VISA resource name out=w710:refnum<visa-resource-name>, error out=w708:errorcluster)  [unwired: 1 out]
                }
                frame "yt" {
                  n235 = local read "pattern"() -> (w717:u32)
                  n236 = VISA Write(VISA resource name=w719, write buffer="s1s", error in (no error)=w718) -> (VISA resource name out=w716:refnum<visa-resource-name>, error out=w715:errorcluster)  [unwired: 1 out]
                  n237 = case shown="9" w717 {
                    tunnel: w716 -> [w722 w726]
                    tunnel: w715 -> [w721 w725]
                    tunnel: [w721 w724] -> w714
                    tunnel: [w722 w723] -> w713
                    frame 0, Default {
                    }
                    frame 9 {
                      n238 = VISA Write(VISA resource name=w726, write buffer="D", error in (no error)=w725) -> (VISA resource name out=w723:refnum<visa-resource-name>, error out=w724:errorcluster)  [unwired: 1 out]
                    }
                  }
                }
                frame "sw" {
                  n239 = local read "pattern"() -> (w728:u32)
                  n240 = case shown="7" w728 {
                    tunnel: w732 -> [w733 w738 w754]
                    tunnel: [w733 w736 w753] -> w731
                    tunnel: w730 -> [w734 w739 w752]
                    tunnel: [w734 w737 w751] -> w729
                    frame 0, Default {
                    }
                    frame 8 {
                      n241 = local read "Sign"() -> (w735:bool)
                      n242 = case shown="False" w735 {
                        tunnel: w738 -> [w741 w748]
                        tunnel: [w740 w747] -> w736
                        tunnel: w739 -> [w743 w746]
                        tunnel: [w742 w745] -> w737
                        frame True {
                          n243 = VISA Write(VISA resource name=w743, write buffer="G", error in (no error)=w741) -> (VISA resource name out=w742:refnum<visa-resource-name>, error out=w740:errorcluster)  [unwired: 1 out]
                        }
                        frame False {
                          n244 = VISA Write(VISA resource name=w746, write buffer="B", error in (no error)=w748) -> (VISA resource name out=w745:refnum<visa-resource-name>, error out=w747:errorcluster)  [unwired: 1 out]
                        }
                      }
                    }
                    frame 7 {
                      n245 = local read "Sign"() -> (w750:bool)
                      n246 = case shown="True" w750 {
                        tunnel: w754 -> [w756 w763]
                        tunnel: [w755 w762] -> w753
                        tunnel: w752 -> [w758 w761]
                        tunnel: [w757 w760] -> w751
                        frame False {
                          n247 = VISA Write(VISA resource name=w758, write buffer="G", error in (no error)=w756) -> (VISA resource name out=w757:refnum<visa-resource-name>, error out=w755:errorcluster)  [unwired: 1 out]
                        }
                        frame True {
                          n248 = VISA Write(VISA resource name=w761, write buffer="B", error in (no error)=w763) -> (VISA resource name out=w760:refnum<visa-resource-name>, error out=w762:errorcluster)  [unwired: 1 out]
                        }
                      }
                    }
                  }
                }
                frame "fs" {
                  n249 = local read "pattern"() -> (w765:u32)
                  n250 = case shown="4" w765 {
                    tunnel: w769 -> [w770 w776 w781 w786 w791]
                    tunnel: [w770 w774 w779 w784 w789] -> w768
                    tunnel: w767 -> [w771 w775 w780 w785 w790]
                    tunnel: [w771 w773 w778 w783 w788] -> w766
                    frame 0, Default {
                    }
                    frame 3 {
                      n251 = VISA Write(VISA resource name=w775, write buffer="s3s", error in (no error)=w776) -> (VISA resource name out=w773:refnum<visa-resource-name>, error out=w774:errorcluster)  [unwired: 1 out]
                    }
                    frame 2 {
                      n252 = VISA Write(VISA resource name=w780, write buffer="s2s", error in (no error)=w781) -> (VISA resource name out=w778:refnum<visa-resource-name>, error out=w779:errorcluster)  [unwired: 1 out]
                    }
                    frame 1 {
                      n253 = VISA Write(VISA resource name=w785, write buffer="s1s", error in (no error)=w786) -> (VISA resource name out=w783:refnum<visa-resource-name>, error out=w784:errorcluster)  [unwired: 1 out]
                    }
                    frame 4 {
                      n254 = VISA Write(VISA resource name=w790, write buffer="s4s", error in (no error)=w791) -> (VISA resource name out=w788:refnum<visa-resource-name>, error out=w789:errorcluster)  [unwired: 1 out]
                    }
                  }
                }
              }
              n255 = feedback #1() -> (w689:errorcluster)  [unwired: 1 in]
              n256 = feedback-in #1(w690) -> ()
              "currentType" <- w682
            }
          }
          n257 = local read "Stop Program"() -> (w643:bool)
          n258 = case shown="Error" w646 {
            selector: w646 -> [_ w678]
            frame No Error {
            }
            frame Error {
              n259 = Unbundle By Name(w678) -> ("source"=w677:string)
              n260 = property on="Stop Program" class="Bool (strict)"("Value"=TRUE) -> ()  [unwired: 2 in, 2 out]
              n261 = One Button Dialog(message=w677) -> ()  [unwired: 1 in, 1 out]
            }
          }
          n262 = Send Notification(notification=w643, notifier=w647, error in (no error)=w646) -> (notifier out=w645:refnum<notifier>, error out=w644:errorcluster)
          n263 = Or(x=w644, y=w643) -> (x .or. y?=w642:bool)
          n264 = Wait (ms)(milliseconds to wait=u32 5) -> ()  [unwired: 1 out]
        }
        n265 = while {
          shift-right: [w483] -> w366
          shift-left: w377 -> [w484]
          shift-right: [w481] -> _
          shift-left: _ -> [w482]
          shift-right: [w479] -> _
          shift-left: u32 0 -> [w478]
          shift-right: [w475] -> _
          shift-left: u8[] [] -> [w476]
          tunnel: w350 -> [w464]
          tunnel: w341 -> [w467]
          tunnel: w334 -> [w466]
          tunnel: [w480] -> w367
          shift-right: [w460] -> _
          shift-left: dbl[] [] -> [w459]
          stop <- w463 stop-if-true
          n266 = Array Size(array=w476) -> (size(s)=w474:i32)
          n267 = Get Notifier Status(notifier=w467, error in (no error)=w466) -> (current notification=w461:bool, error out=w462:errorcluster)  [unwired: 3 out]
          n268 = Or(x=w462, y=w461) -> (x .or. y?=w463:bool)
          n269 = Dequeue Element(queue=w464, timeout in ms (-1)=250, error in (no error)=w462) -> (element=w471:u8[], error out=w468:errorcluster)  [unwired: 2 out]
          n270 = Insert Into Array(array=w476, index=w474, new element=w471) -> (w470:u8[])
          n271 = Array Size(array=w470) -> (size(s)=w469:i32)
          n272 = Greater?(x=w469, y=0) -> (0:w472:bool)
          n273 = case shown="True" w472 {
            tunnel: w468 -> [w490 w526]
            tunnel: [w490 w570] -> w480
            tunnel: w484 -> [w489 w532]
            tunnel: [w489 w569] -> w483
            tunnel: [w488 w499] -> w481
            tunnel: w482 -> [w488 w527]
            tunnel: [w487 w513] -> w479
            tunnel: w478 -> [w487 w514]
            tunnel: w470 -> [w486 w508]
            tunnel: [w486 w505] -> w475
            tunnel: [w485 w495] -> w460
            tunnel: w459 -> [w485 w501]
            frame False {
            }
            frame True {
              n274 = flat-sequence {
                tunnel: [w631] -> w568
                tunnel: [w630] -> w515
                tunnel: w568 -> [w634]
                tunnel: w515 -> [w635]
                tunnel: [w637] -> w513
                tunnel: w514 -> [w636]
                frame #0 {
                  n275 = local read "millisecond timer value 2"() -> (w632:u32)
                  n276 = Tick Count (ms)() -> (millisecond timer value=w631:u32)
                  n277 = Subtract(x=w631, y=w632) -> (x-y=w630:u32)
                  "Timing" <- w630
                }
                frame #1 {
                  n278 = Not Equal?(x=w634, y=w635) -> (x != y?=w633:bool)
                  n279 = local write "millisecond timer value 2"(w634) -> ()
                  n280 = case shown="True" w633 {
                    tunnel: w635 -> [_ w641]
                    tunnel: [u32 0 w640] -> w637
                    tunnel: w636 -> [_ w639]
                    frame False {
                    }
                    frame True {
                      n281 = Add(x=w641, y=w639) -> (x+y=w640:u32)
                    }
                  }
                }
              }
              n282 = Get File Size(file=w532, error in=w526) -> (refnum out=w575:refnum<file>, size (in bytes)=w574:i64, 0:w573:errorcluster)
              n283 = Delete From Array(array=w508, length=4, index=0) -> (deleted portion=w504:u8[], array with subset deleted=w505:u8[])
              n284 = Set File Position(offset (in bytes) (0)=w574, refnum=w575, error in=w573) -> (refnum out=w571:refnum<file>, error out=w572:errorcluster)  [unwired: 1 in]
              n285 = Index Array(array=w504, index=2) -> (element=w529:u8)
              n286 = Index Array(array=w504, index=3) -> (element=w528:u8)
              n287 = Index Array(array=w504, index=0) -> (element=w531:u8)
              n288 = Index Array(array=w504, index=1) -> (element=w530:u8)
              n289 = Number To Boolean Array(number=w529) -> (Boolean array=w550:bool[])
              n290 = Number To Boolean Array(number=w528) -> (Boolean array=w553:bool[])
              n291 = Number To Boolean Array(number=w531) -> (Boolean array=w540:bool[])
              n292 = Number To Boolean Array(number=w530) -> (Boolean array=w559:bool[])
              n293 = Index Array(array=w559, index=5) -> (element=w561:bool)
              n294 = Delete From Array(array=w550, length=2, index=6 ("length")) -> (array with subset deleted=w563:bool[])  [unwired: 1 out]
              n295 = Delete From Array(array=w553, length=2, index=6) -> (array with subset deleted=w564:bool[])  [unwired: 1 out]
              n296 = Delete From Array(array=w540, length=2, index=6 ("length")) -> (array with subset deleted=w543:bool[])  [unwired: 1 out]
              n297 = Delete From Array(array=w559, length=3, index=5) -> (array with subset deleted=w548:bool[])  [unwired: 1 out]
              n298 = Insert Into Array(array=w563, index=6, new element=w564) -> (w557:bool[])
              n299 = Insert Into Array(array=w543, index=6, new element=w548) -> (w545:bool[])
              n300 = case shown="True" w561 {
                tunnel: w545 -> [w622 w629]
                tunnel: [w622 w624] -> w562
                frame False {
                }
                frame True {
                  n301 = Build Array (concatenate)(w629, TRUE ("new element/subarray"), TRUE ("new element/subarray"), TRUE ("new element/subarray"), TRUE ("new element/subarray"), TRUE ("element")) -> (w624:bool[])
                }
              }
              n302 = Boolean Array To Number(Boolean array=w557) -> (number=w558:u32)
              n303 = To Unsigned Word Integer(number=w558) -> (unsigned 16bit integer=w499:u16)
              "Int_pixel" <- w499
              n304 = Boolean Array To Number(Boolean array=w562) -> (number=w549:u32)
              n305 = To Word Integer(number=w549) -> (16bit integer=w509:i16)
              "AD_Value" <- w509
              n306 = local read "contingency"() -> (w516:string)
              n307 = Subtract(x=w499, y=w527) -> (x-y=→"x-y":u16)
              n308 = To Double Precision Float(number=w499) -> (double precision float=w500:dbl)
              n309 = Multiply(x=w499, y=4.5) -> (x*y=w518:dbl)
              n310 = local read "Timeslot"() -> (w522:i32)
              n311 = case shown="\"left_torque\"" w516 {
                tunnel: w499 -> [_ w580 w606 _ _]
                tunnel: w509 -> [_ _ _ w612 w617]
                frame "False", Default {
                  n312 = local write "PWM"(FALSE ("pwm")) -> ()
                }
                frame "1_3_Q" {
                  n313 = Greater Or Equal?(x=w580, y=u16 0 ("x")) -> (x >= y?=w579:bool)
                  n314 = Less?(x=w580, y=u16 100) -> (x < y?=w590:bool)
                  n315 = Greater?(x=w580, y=u16 300 ("a")) -> (0:w592:bool)
                  n316 = Less?(x=w580, y=u16 500 ("b")) -> (x < y?=w591:bool)
                  n317 = Greater?(x=w580, y=u16 700) -> (0:w589:bool)
                  n318 = Less Or Equal?(x=w580, y=u16 799) -> (x <= y?=w587:bool)
                  n319 = And(x=w579, y=w590) -> (x .and. y?=w585:bool)
                  n320 = And(x=w592, y=w591) -> (x .and. y?=w584:bool)
                  n321 = And(x=w589, y=w587) -> (x .and. y?=w583:bool)
                  n322 = Compound Arithmetic op=OR(w585, w584, w583) -> (w582:bool)
                  n323 = case shown="True" w582 {
                    frame False {
                      n324 = local write "PWM"(FALSE ("pwm")) -> ()
                    }
                    frame True {
                      n325 = local write "PWM"(TRUE ("pwm")) -> ()
                    }
                  }
                }
                frame "2_4_Q" {
                  n326 = Greater?(x=w606, y=u16 100 ("x")) -> (0:w601:bool)
                  n327 = Less?(x=w606, y=u16 300) -> (x < y?=w602:bool)
                  n328 = Greater?(x=w606, y=u16 500 ("a")) -> (0:w605:bool)
                  n329 = Less?(x=w606, y=u16 700 ("b")) -> (x < y?=w603:bool)
                  n330 = And(x=w601, y=w602) -> (x .and. y?=w600:bool)
                  n331 = And(x=w605, y=w603) -> (x .and. y?=w604:bool)
                  n332 = Or(x=w600, y=w604) -> (x .or. y?=w599:bool)
                  n333 = case shown="True" w599 {
                    frame False {
                      n334 = local write "PWM"(FALSE ("pwm")) -> ()
                    }
                    frame True {
                      n335 = local write "PWM"(TRUE ("pwm")) -> ()
                    }
                  }
                }
                frame "right_torque" {
                  n336 = Greater Or Equal?(x=w612, y=i16 0) -> (x >= y?=w613:bool)
                  n337 = case shown="True" w613 {
                    frame False {
                      n338 = local write "PWM"(TRUE ("pwm")) -> ()
                    }
                    frame True {
                      n339 = local write "PWM"(FALSE ("pwm")) -> ()
                    }
                  }
                }
                frame "left_torque" {
                  n340 = Greater Or Equal?(x=w617, y=i16 0) -> (x >= y?=w618:bool)
                  n341 = case shown="True" w618 {
                    frame False {
                      n342 = local write "PWM"(FALSE ("pwm")) -> ()
                    }
                    frame True {
                      n343 = local write "PWM"(TRUE ("pwm")) -> ()
                    }
                  }
                }
              }
              n344 = To Long Integer(number=w518) -> (32bit integer=w517:i32)
              n345 = To Long Integer(number=w509) -> (32bit integer=w520:i32)
              n346 = Bundle(w499, w509) -> (→"Kombi Chart":cluster{u16, i16})  [unwired: 1 in]
              n347 = Greater Or Equal?(x=w509, y=i16 0) -> (x >= y?=w510:bool)
              n348 = case shown="False" w510 {
                frame False {
                  n349 = local write "Sign"(FALSE) -> ()
                }
                frame True {
                  n350 = local write "Sign"(TRUE) -> ()
                }
              }
              n351 = Insert Into Array(array=w501, index=0, new element=w500) -> (w495:dbl[])
              n352 = Number To Decimal String(number=w513) -> (decimal integer string=w525:string)  [unwired: 1 in]
              n353 = Number To Decimal String(number=w517) -> (decimal integer string=w565:string)  [unwired: 1 in]
              n354 = Number To Decimal String(number=w520) -> (decimal integer string=w523:string)  [unwired: 1 in]
              n355 = Number To Decimal String(number=w522) -> (decimal integer string=w521:string)  [unwired: 1 in]
              n356 = Array Size(array=w495) -> (size(s)=w494:i32)
              n357 = call <vilib>:"General Histogram.vi"("X"=w495, "max"=800.0, "min"=0.0, "# bins"=10) -> ("Histogram"=w493:i32[], "Axis"=w496:dbl[])  [unwired: 7 in, 3 out]
              n358 = Concatenate Strings(w525, "\t" ("string"), w565, "\t" ("string"), w523, "\t" ("string"), w521, "\r\n") -> (w533:string)
              n359 = Divide(x=w493, y=w494) -> (x/y=w492:dbl[])
              n360 = Bundle("Axis"=w496, w492) -> (→"Histogram Graph":cluster{"Axis":dbl[], dbl[]})  [unwired: 1 in]
              n361 = Write to Text File(file (use dialog)=w571, text=w533, error in=w572) -> (refnum out=w569:refnum<file>, error out=w570:errorcluster)  [unwired: 1 in, 1 out]
            }
          }
          n362 = Wait (ms)(milliseconds to wait=u32 5) -> ()  [unwired: 1 out]
        }
        n363 = while {
          tunnel: w398 -> [w426]
          tunnel: w334 -> [w425]
          shift-right: [w423] -> _
          shift-left: FALSE ("pwm") -> [w427]
          tunnel: [w424] -> w383
          tunnel: [w416] -> w405
          stop <- w417 stop-if-true
          n364 = local read "outcome"() -> (w422:u32)
          n365 = Not Equal?(x=w422, y=u32 0) -> (x != y?=w420:bool)
          n366 = case shown="True" w420 {
            tunnel: w427 -> [w430 w449]
            tunnel: w426 -> [w434 w444]
            tunnel: w425 -> [w432 w445]
            tunnel: [w433 w448] -> w424
            tunnel: [w431 w447] -> w416
            tunnel: [w429 w446] -> w423
            frame False {
              w429 = FALSE ("Boolean")
              n367 = Not Equal?(x=w429, y=w430) -> (x != y?=w428:bool)
              n368 = case shown="True" w428 {
                tunnel: w434 -> [w436 w442]
                tunnel: [w436 w441] -> w433
                tunnel: w432 -> [w435 w440]
                tunnel: [w435 w439] -> w431
                frame False {
                }
                frame True {
                  n369 = call "labjack.vi"("error out"=w440, "Boolean"=FALSE, "Handle Out"=w442) -> ("error out 2"=w439:errorcluster, "Boolean 2"=w437:bool, "Handle Out 2"=w441:i32)  [unwired: 6 in]
                  n370 = local write "Output"(w437) -> ()
                }
              }
            }
            frame True {
              n371 = local read "PWM"() -> (w446:bool)
              n372 = Not Equal?(x=w449, y=w446) -> (x != y?=w443:bool)
              n373 = case shown="True" w443 {
                tunnel: w444 -> [w451 w458]
                tunnel: w445 -> [w450 w457]
                tunnel: [w451 w456] -> w448
                tunnel: [w450 w455] -> w447
                frame False {
                }
                frame True {
                  n374 = local read "PWM"() -> (w454:bool)
                  n375 = call "labjack.vi"("error out"=w457, "PwmDtc"="pwmDtc", "Boolean"=w454, "Handle Out"=w458) -> ("error out 2"=w455:errorcluster, "Boolean 2"=w453:bool, "Handle Out 2"=w456:i32)  [unwired: 5 in]
                  n376 = local write "Output"(w453) -> ()
                }
              }
            }
          }
          n377 = Wait (ms)(milliseconds to wait=u32 5) -> ()  [unwired: 1 out]
          n378 = local read "Stop Program"() -> (w418:bool)
          n379 = Or(x=w416, y=w418) -> (x .or. y?=w417:bool)
        }
        n380 = Merge Errors(w338, w367, w405) -> (w337:errorcluster)
        n381 = Release Queue(queue=w349, error in (no error)=w337) -> (error out=w340:errorcluster)  [unwired: 1 in, 2 out]
        n382 = Release Notifier(notifier=w339, error in (no error)=w340) -> (error out=w336:errorcluster)  [unwired: 1 in, 2 out]
        n383 = VISA Write(VISA resource name=w359, write buffer="S", error in (no error)=w336) -> (VISA resource name out=w358:refnum<visa-resource-name>, error out=w360:errorcluster)  [unwired: 1 out]
        n384 = Close File(refnum=w366, error in=w360) -> (error out=w365:errorcluster)  [unwired: 1 out]
        n385 = call "rename_xml.vi"("error in"=w365, "xml"=w328, "csv"=w363) -> ("error out"=w364:errorcluster)  [unwired: 4 in]
        n386 = VISA Close(VISA resource name=w358, error in (no error)=w364) -> (error out=w388:errorcluster)
        n387 = call "labjack.vi"("error out"=w388, "Boolean"=FALSE, "Handle Out"=w383) -> ("error out 2"=w389:errorcluster, "Handle Out 2"=w387:i32)  [unwired: 6 in, 1 out]
        n388 = call "LJM_Close.vi"("error in"=w389, "Handle"=w387) -> ("error out"=w386:errorcluster)  [unwired: 9 in]
        "error out" <- w386
        n389 = call "LJM_ErrorToString.vi"("error in"=w386) -> ("String"=→"Error String":string)  [unwired: 10 in]
      }
    }
    n390 = local write "millisecond timer value 2"("millisecond timer value 2") -> ()
    n391 = Wait (ms)(milliseconds to wait=u32 5) -> ()  [unwired: 1 out]
    n392 = local read "Stop Program"() -> (w320:bool)
  }
  n393 = flat-sequence {
    tunnel: w17 -> [w851]
    tunnel: [w851] -> w16
    tunnel: w16 -> [w852]
    frame #0 {
      n394 = Not(x=w851) -> (.not. x?=w850:bool)
      n395 = local write "Stop Program"(w850) -> ()
    }
    frame #1 {
      n396 = Stop(stop? (T)=w852) -> ()
    }
  }
  "Progress" <- 0.0 ("Slide")
  "Time" <- 0.0 ("Progress 2")
